vi "pwm speed.vi"(5 "PWM":cluster{"divider":i32, "period":i32}, 7 "motor  ?":enum16{"M1", "M2", "M3", "M4"}(ring), 8 "error in":errorcluster, 9 "brake":bool, 10 "speed":dbl, 11 "FPGA VI Reference":refnum<k20>) -> (0 "error out":errorcluster, 3 "FPGA VI Reference Out":refnum<k20>)   [LabVIEW 2019, in "my FPGA lib.lvlib" / "motor.lvclass"]
uses:
  motor.lvclass
  <vilib>/Utility/error.llb/Error Cluster From Error Code.vi
  <vilib>/rvi/errors/niLvFpgaAdjustHostInterfaceError.vi
  <vilib>/rvi/interface/nirviReadWriteControl/nirviReadWriteControl.xnode
  NiFpgaLv.dll
  <vilib>/rvi/interface/Simulation/niFpgaSimulationCallBeginRW.vi
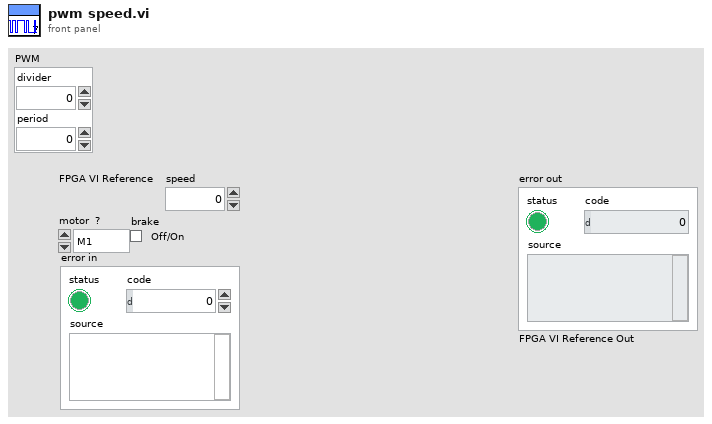
[diagram p1: front panel]
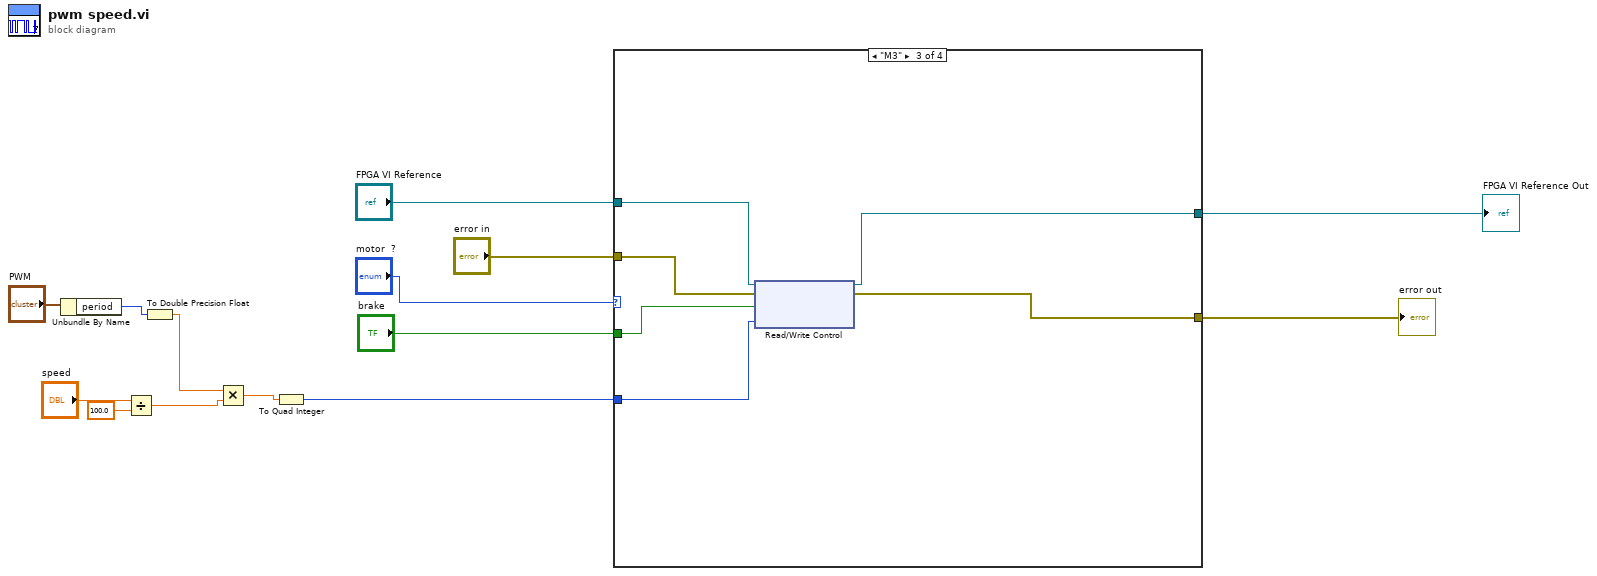
[diagram p0: block diagram]
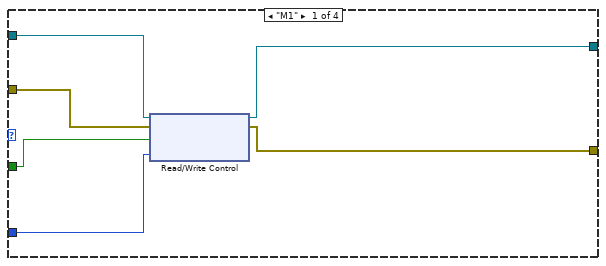
[diagram p2: hidden frame]
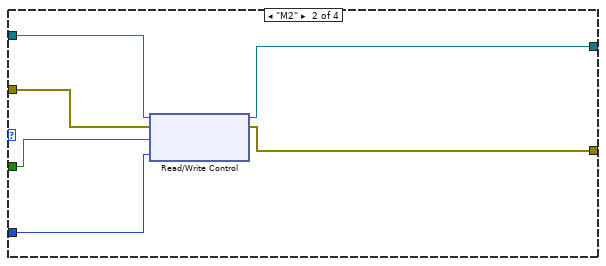
[diagram p3: hidden frame]
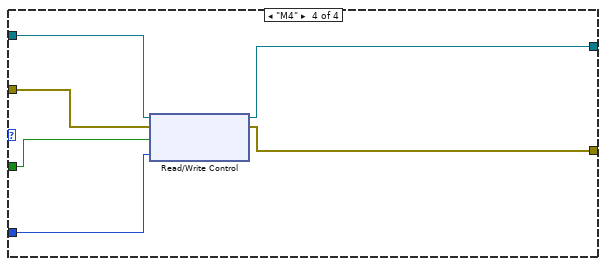
[diagram p4: hidden frame]
diagram:
  n1 = Unbundle By Name("PWM") -> ("period"=w4:i32)
  n2 = Divide(x="speed", y=100.0) -> (x/y=w5:dbl)
  n3 = To Double Precision Float(number=w4) -> (double precision float=w3:dbl)
  n4 = Multiply(x=w3, y=w5) -> (x*y=w2:dbl)
  n5 = To Quad Integer(1:w2) -> (0:w1:i64)
  n6 = case shown="\"M3\"" "motor  ?" {
    tunnel: "FPGA VI Reference" -> [w20 w26 w32 w38]
    tunnel: "error in" -> [w19 w25 w31 w37]
    tunnel: "brake" -> [w17 w24 w30 w35]
    tunnel: w1 -> [w18 w23 w29 w36]
    tunnel: [w16 w21 w27 w33] -> w10
    tunnel: [w15 w22 w28 w34] -> w9
    frame "M1" {
      n7 = xnode "Read/Write Control"("FPGA VI Reference In"=w20, "error in"=w19, "Motor1.brake"=w17, "Motor1.speed"=w18) -> ("FPGA VI Reference Out"=w15:refnum<k20>, "error out"=w16:errorcluster)
    }
    frame "M2" {
      n8 = xnode "Read/Write Control"("FPGA VI Reference In"=w26, "error in"=w25, "Motor2.brake"=w24, "Motor2.speed"=w23) -> ("FPGA VI Reference Out"=w22:refnum<k20>, "error out"=w21:errorcluster)
    }
    frame "M3" {
      n9 = xnode "Read/Write Control"("FPGA VI Reference In"=w32, "error in"=w31, "Motor3.brake"=w30, "Motor3.speed"=w29) -> ("FPGA VI Reference Out"=w28:refnum<k20>, "error out"=w27:errorcluster)
    }
    frame "M4" {
      n10 = xnode "Read/Write Control"("FPGA VI Reference In"=w38, "error in"=w37, "Motor4.brake"=w35, "Motor4.speed"=w36) -> ("FPGA VI Reference Out"=w34:refnum<k20>, "error out"=w33:errorcluster)
    }
  }
  "error out" <- w10
  "FPGA VI Reference Out" <- w9
